vi "Query Buffer.vi"(8 "error in (no error)":errorcluster, 11 "VISA resource name":refnum<visa-resource-name>) -> (0 "error out":errorcluster, 1 "appended array":dbl[](array[numeric]), 3 "VISA resource name out":refnum<visa-resource-name>)   [LabVIEW 2015, in "SR400.lvlib"]
uses:
  SR400.lvlib
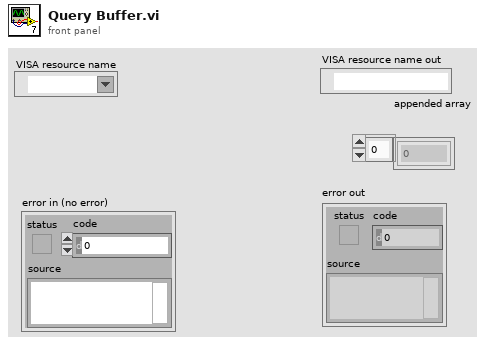
[diagram p1: front panel]
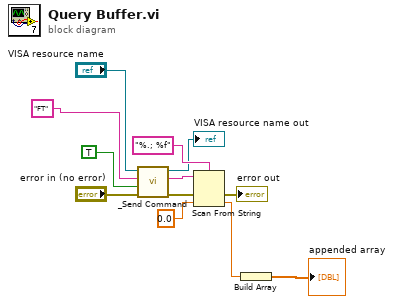
[diagram p0: block diagram]
diagram:
  n1 = call "_Send Command.vi"("error in (no error)"="error in (no error)", "Query? (F)"=TRUE, "Command"="FT", "VISA resource name"="VISA resource name") -> ("error out"=w5:errorcluster, "Response"=w6:string, "VISA resource name out"=→"VISA resource name out":refnum<visa-resource-name>)  [unwired: 5 out]
  n2 = Scan From String(format string="%.; %f", input string=w6, error in=w5, default 1=0.0 ("default value 1")) -> (error out=→"error out":errorcluster, output 1=w2:dbl)  [unwired: 1 in, 2 out]
  n3 = Build Array(w2) -> (→"appended array":dbl[])
